vi "uTTA_SendQuery.vi"(4 "RX Termination(\\n)":string="\n", 6 "Timeout(ms)":i32=1000, 7 "Send String":string, 8 "error in (no error)":errorcluster, 10 "TX Termination(\\n)":string="\n", 11 "VISA Refnum in":refnum<visa-resource-name>) -> (0 "error out":errorcluster, 2 "Received":string, 3 "VISA Refnum out":refnum<visa-resource-name>)   [LabVIEW 2021]
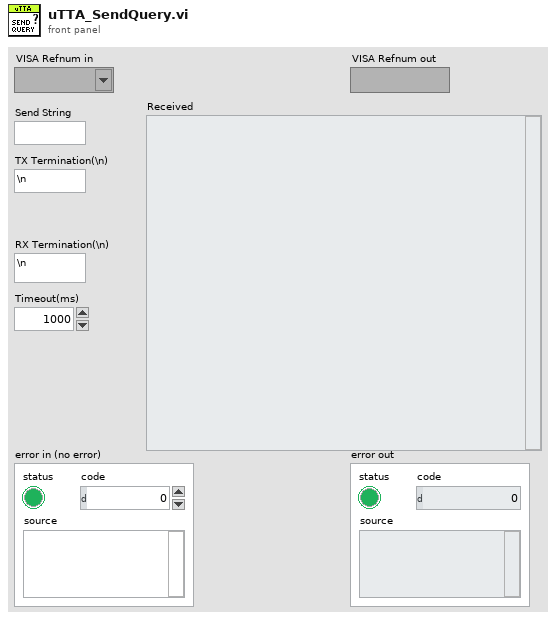
[diagram p1: front panel]
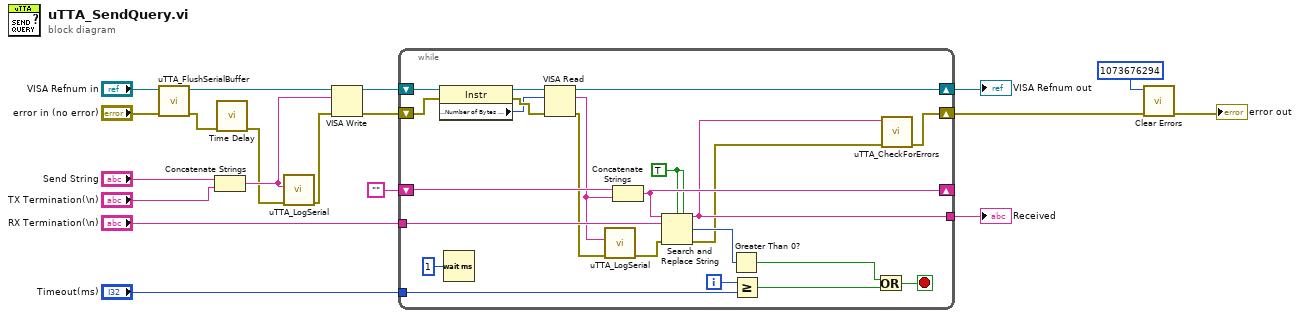
[diagram p0: block diagram]
diagram:
  n1 = call "uTTA_FlushSerialBuffer.vi"("error in (no error)"="error in (no error)", "VISA Refnum in"="VISA Refnum in") -> ("error out"=w3:errorcluster, "VISA Refnum out"=w4:refnum<visa-resource-name>)  [unwired: 4 in]
  n2 = Concatenate Strings("Send String", "TX Termination(\\n)") -> (w7:string)
  n3 = call "Time Delay"("error in (no error)"=w3) -> ("error out"=w2:errorcluster)  [unwired: 10 in]
  n4 = call "uTTA_LogSerial.vi"("error in"=w2, "Data_Sent"=w7) -> ("error out"=w1:errorcluster)  [unwired: 5 in]
  n5 = VISA Write(VISA resource name=w4, write buffer=w7, error in (no error)=w1) -> (VISA resource name out=w13:refnum<visa-resource-name>, error out=w14:errorcluster)  [unwired: 1 out]
  n6 = while {
    shift-right: [w36] -> _
    shift-left: "" -> [w37]
    tunnel: [w26] -> w9
    shift-right: [w24] -> w11
    shift-left: w14 -> [w41]
    shift-right: [w33] -> w18
    shift-left: w13 -> [w42]
    tunnel: "Timeout(ms)" -> [w28]
    tunnel: "RX Termination(\\n)" -> [w27]
    i -> [w29]
    stop <- w31 stop-if-true
    w23 = TRUE ("ignore case? (F)")
    n7 = property class="Instr"(reference=w42, error in=w41) -> (reference out=w40:refnum<visa-resource-name>, error out=w39:errorcluster, "Serial Settings:Number of Bytes at Serial Port"=w38:u32)
    n8 = Wait (ms)(milliseconds to wait=u32 1) -> ()  [unwired: 1 out]
    n9 = VISA Read(VISA resource name=w40, byte count=w38, error in (no error)=w39) -> (VISA resource name out=w33:refnum<visa-resource-name>, read buffer=w22:string, error out=w21:errorcluster)  [unwired: 1 out]
    n10 = call "uTTA_LogSerial.vi"("error in"=w21, "Data_Sent"=w22) -> ("error out"=w20:errorcluster)  [unwired: 5 in]
    n11 = Concatenate Strings(w37, w22) -> (w36:string)
    n12 = Search and Replace String(case sensitive?=w23, multiline?=w23, input string=w36, search string=w27, error in=w20) -> (result string=w26:string, number of replacements=w35:i32, error out=w25:errorcluster)  [unwired: 3 in, 1 out]
    n13 = Greater Than 0?(x=w35) -> (x > 0?=w32:bool)
    n14 = Greater Or Equal?(x=w29, y=w28) -> (x >= y?=w30:bool)
    n15 = Or(x=w32, y=w30) -> (x .or. y?=w31:bool)
    n16 = call "uTTA_CheckForErrors.vi"("error in"=w25, "Received"=w26) -> ("error out"=w24:errorcluster)  [unwired: 9 in]
  }
  "Received" <- w9
  "VISA Refnum out" <- w18
  n17 = call <vilib>:"Clear Errors.vi"("error in (no error)"=w11, "specific error code to clear (0: all)"=1073676294) -> ("error out"=→"error out":errorcluster)  [unwired: 4 in, 1 out]
